vi "initFPObjectsMain.vi"(8 "error in (no error)":errorcluster {"code" format="Error %.0f"}, 11 "mainRefs":T1) -> (0 "error out":errorcluster {"code" format="Error %.0f"})   [LabVIEW 2017]
doc: "This VI uses the FP object rest to define and set the default value adn state for startup/shutdown."
uses:
  Controls/objectRefsMain.ctl
  globalConstants.vi
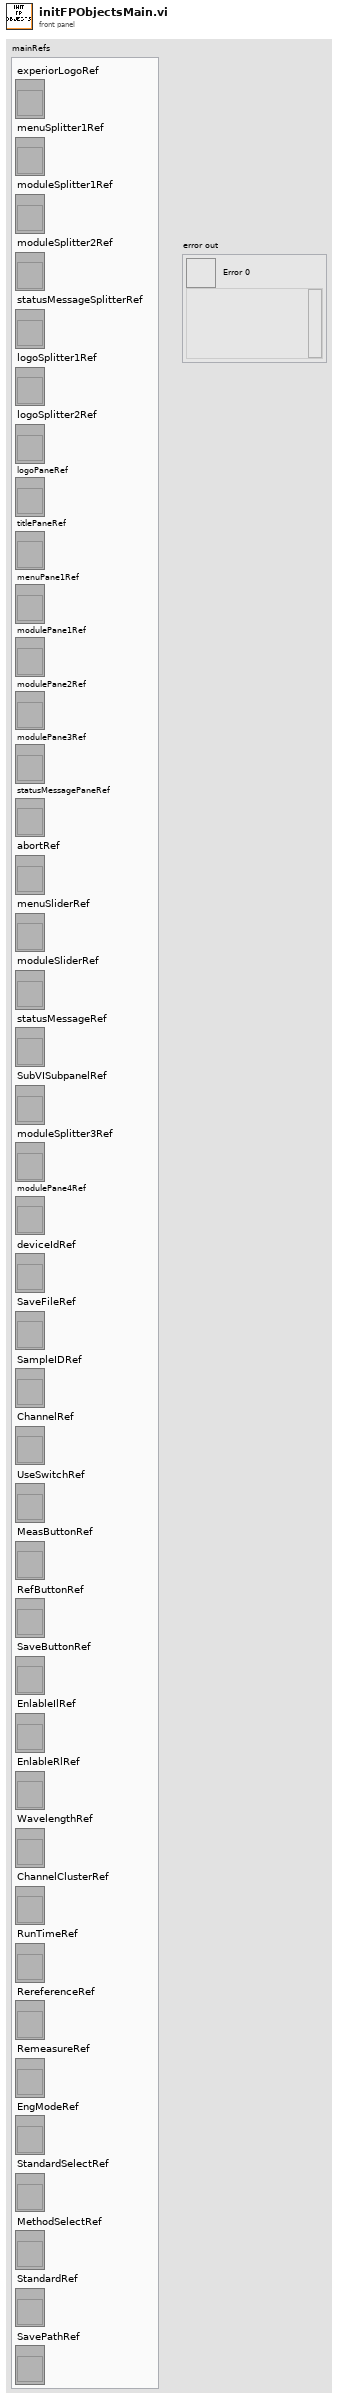
[diagram p1: front panel]
types:
  T1 = typedef "objectRefsMain.ctl" = cluster{"experiorLogoRef":refnum<vi>, "menuSplitter1Ref":refnum<vi>, "moduleSplitter1Ref":refnum<vi>, "moduleSplitter2Ref":refnum<vi>, "statusMessageSplitterRef":refnum<vi>, "logoSplitter1Ref":refnum<vi>, "logoSplitter2Ref":refnum<vi>, "logoPaneRef":refnum<vi>, "titlePaneRef":refnum<vi>, "menuPane1Ref":refnum<vi>, "modulePane1Ref":refnum<vi>, "modulePane2Ref":refnum<vi>, "modulePane3Ref":refnum<vi>, "statusMessagePaneRef":refnum<vi>, "abortRef":refnum<vi>, "menuSliderRef":refnum<vi>, "moduleSliderRef":refnum<vi>, "statusMessageRef":refnum<vi>, "SubVISubpanelRef":refnum<vi>, "moduleSplitter3Ref":refnum<vi>, "modulePane4Ref":refnum<vi>, "deviceIdRef":refnum<vi>, "SaveFileRef":refnum<vi>, "SampleIDRef":refnum<vi>, "ChannelRef":refnum<vi>, "UseSwitchRef":refnum<vi>, "MeasButtonRef":refnum<vi>, "RefButtonRef":refnum<vi>, "SaveButtonRef":refnum<vi>, "EnlableIlRef":refnum<vi>, "EnlableRlRef":refnum<vi>, "WavelengthRef":refnum<vi>, "ChannelClusterRef":refnum<vi>, "RunTimeRef":refnum<vi>, "RereferenceRef":refnum<vi>, "RemeasureRef":refnum<vi>, "EngModeRef":refnum<vi>, "StandardSelectRef":refnum<vi>, "MethodSelectRef":refnum<vi>, "StandardRef":refnum<vi>, "SavePathRef":refnum<vi>}
  T2 = enum16{"No Scaling", "Scale All Objects", "Scale Single Object"}
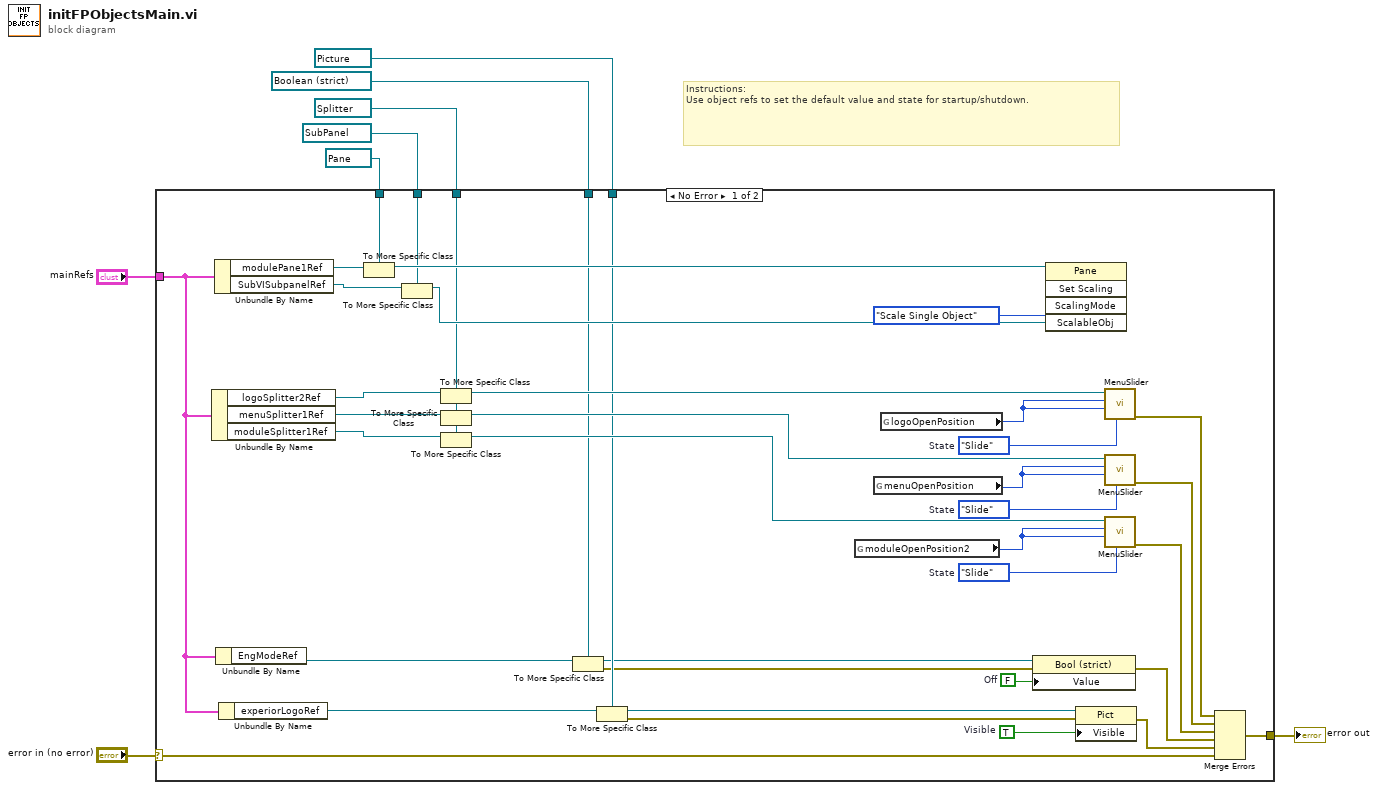
[diagram p0: block diagram]
diagram:
  # "Instructions:\nUse object refs to set the default value and state for startup/shutdown."
  n1 = case shown="No Error" "error in (no error)" {
    selector: "error in (no error)" -> [w39 w47]
    tunnel: [w44 w47] -> w7
    tunnel: "mainRefs" -> [w10 _]
    tunnel: refnum<vi> refnum ("logoPaneRef") -> [w45 _]
    tunnel: refnum<vi> refnum ("logoPaneRef") -> [w40 _]
    tunnel: refnum<vi> refnum ("logoPaneRef") -> [w27 _]
    tunnel: refnum<vi> refnum ("logoPaneRef") -> [w23 _]
    tunnel: refnum<vi> refnum ("Enable IL") -> [w12 _]
    frame No Error {
      w16 = FALSE  # Off
      w21 = TRUE  # Visible
      w32 = enum16{"Reset", "Slide"}."Slide"  # State
      w33 = enum16{"Reset", "Slide"}."Slide"  # State
      w35 = enum16{"Reset", "Slide"}."Slide"  # State
      n2 = Unbundle By Name(w10) -> ("logoSplitter2Ref"=w37:refnum<vi>, "menuSplitter1Ref"=w29:refnum<vi>, "moduleSplitter1Ref"=w28:refnum<vi>)
      n3 = Unbundle By Name(w10) -> ("modulePane1Ref"=w46:refnum<vi>, "SubVISubpanelRef"=w41:refnum<vi>)
      n4 = Unbundle By Name(w10) -> ("EngModeRef"=w15:refnum<vi>)
      n5 = Unbundle By Name(w10) -> ("experiorLogoRef"=w24:refnum<vi>)
      n6 = To More Specific Class(target class=w45, reference=w46) -> (specific class reference=w43:refnum<vi>)  [unwired: 1 in, 1 out]
      n7 = To More Specific Class(target class=w40, reference=w41) -> (specific class reference=w38:refnum<vi>)  [unwired: 1 in, 1 out]
      n8 = To More Specific Class(target class=w27, reference=w37) -> (specific class reference=w36:refnum<vi>)  [unwired: 1 in, 1 out]
      n9 = To More Specific Class(target class=w27, reference=w29) -> (specific class reference=w26:refnum<vi>)  [unwired: 1 in, 1 out]
      n10 = To More Specific Class(target class=w27, reference=w28) -> (specific class reference=w25:refnum<vi>)  [unwired: 1 in, 1 out]
      n11 = To More Specific Class(target class=w12, reference=w15) -> (specific class reference=w14:refnum<vi>, error out=w13:errorcluster)  [unwired: 1 in]
      n12 = To More Specific Class(target class=w23, reference=w24) -> (specific class reference=w22:refnum<vi>, error out=w11:errorcluster)  [unwired: 1 in]
      n13 = global read "globalConstants.vi" "moduleOpenPosition2"() -> (w30:u32)
      n14 = global read "globalConstants.vi" "menuOpenPosition"() -> (w31:u32)
      n15 = global read "globalConstants.vi" "logoOpenPosition"() -> (w34:u32)
      n16 = property class="Bool (strict)"(reference=w14, error in=w13, "Value"=w16) -> (error out=w9:errorcluster)  [unwired: 1 out]
      n17 = invoke class="Pane" method="Set Scaling"(reference=w43, "ScalingMode"=T2."Scale Single Object" ("Scaling Mode"), "ScalableObj"=w38) -> ()  [unwired: 2 in, 5 out]
      n18 = property class="Pict"(reference=w22, error in=w11, "Visible"=w21) -> (error out=w20:errorcluster)  [unwired: 1 out]
      n19 = call "MenuSlider.vi"("State"=w35, "Open Position"=w34, "Close Position"=w34, "Splitter Refnum"=w36) -> ("Error Out"=w17:errorcluster)  [unwired: 7 in]
      n20 = call "MenuSlider.vi"("State"=w33, "Open Position"=w31, "Close Position"=w31, "Splitter Refnum"=w26) -> ("Error Out"=w18:errorcluster)  [unwired: 7 in]
      n21 = call "MenuSlider.vi"("State"=w32, "Open Position"=w30, "Close Position"=w30, "Splitter Refnum"=w25) -> ("Error Out"=w19:errorcluster)  [unwired: 7 in]
      n22 = Merge Errors(w17, w18, w19, w9, w20, w39) -> (w44:errorcluster)
    }
    frame Error {
    }
  }
  "error out" <- w7
